vi "Decrease Loop Delay.vi"(8 "Amount to Decrease":u32=2, 10 "Y Hit Lower Boundary?":bool, 11 "Current Delay":u32) -> (3 "Next Delay":u32)   [LabVIEW 2015]
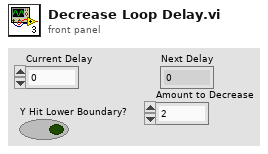
[diagram p1: front panel]
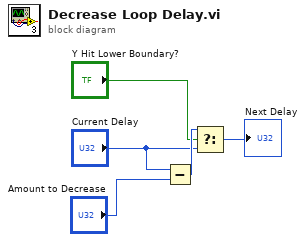
[diagram p0: block diagram]
diagram:
  n1 = Subtract(x="Current Delay", y="Amount to Decrease") -> (x-y=w3:u32)
  n2 = Select(t=w3, s="Y Hit Lower Boundary?", f="Current Delay") -> (s? t:f=→"Next Delay":u32)
